vi "Credito de Monedas.vi"(8 "error in (no error)":errorcluster, 10 "Dinero":i32, 11 "Monedas in":refnum<class "Monedas.lvclass">) -> (0 "error out":errorcluster, 3 "Monedas out":refnum<class "Monedas.lvclass">)   [LabVIEW 2020, in "Monedas.lvlib" / "Monedas.lvclass"]
uses:
  Monedas.lvclass
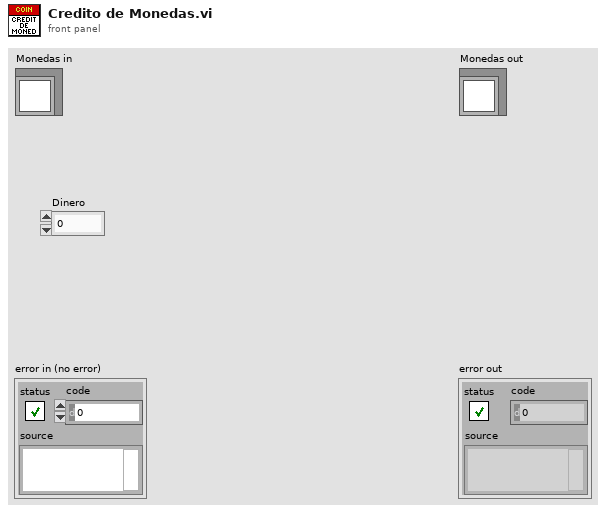
[diagram p1: front panel]
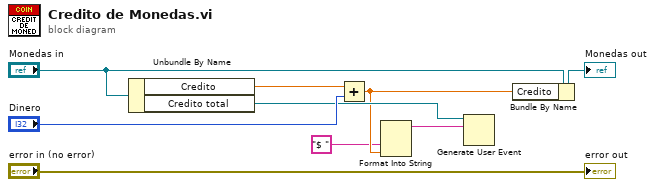
[diagram p0: block diagram]
diagram:
  n1 = Unbundle By Name("Monedas in") -> ("Credito"=w5:dbl, "Credito total"=w3:refnum<user-event>)
  n2 = Add(x=w5, y="Dinero") -> (x+y=w2:dbl)
  n3 = Format Into String("$ ", w2) -> (resulting string=w4:string)  [unwired: 3 in, 1 out]
  n4 = Generate User Event(user event=w3, event data cluster=w4) -> ()  [unwired: 2 in, 2 out]
  n5 = Bundle By Name(cluster="Monedas in", "Credito"=w2) -> (→"Monedas out":refnum<class "Monedas.lvclass">)
  "error out" <- "error in (no error)"
